vi "Error log.vi"(8 "error in (no error)":errorcluster) -> ()   [LabVIEW 2020]
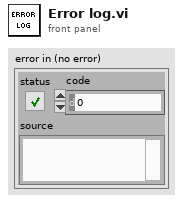
[diagram p1: front panel]
types:
  T1 = enum16{"open", "replace", "create", "open or create", "replace or create", "replace or create with confirmation"}
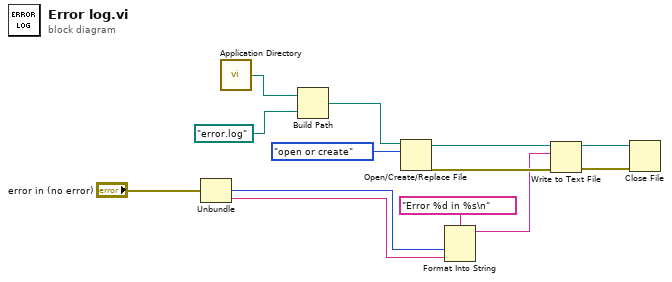
[diagram p0: block diagram]
diagram:
  n1 = Unbundle("error in (no error)") -> ("code"=w8:i32, "source"=w7:string)  [unwired: 1 out]
  n2 = call <vilib>:"Application Directory.vi"() -> ("Application Directory"=w11:path)
  n3 = Build Path(base path=w11, name or relative path=path "error.log") -> (appended path=w10:path)
  n4 = Open/Create/Replace File(file path (use dialog)=w10, operation (0:open)=T1."open or create") -> (refnum out=w4:refnum<file>, error out=w5:errorcluster)  [unwired: 4 in, 1 out]
  n5 = Format Into String(format string="Error %d in %s\n", w8, w7) -> (resulting string=w3:string)  [unwired: 2 in, 1 out]
  n6 = Write to Text File(file (use dialog)=w4, text=w3, error in=w5) -> (refnum out=w1:refnum<file>, error out=w2:errorcluster)  [unwired: 1 in, 1 out]
  n7 = Close File(refnum=w1, error in=w2) -> ()  [unwired: 2 out]
